vi "GetIQ_sglwfm.vi"(8 "error in (no error)":errorcluster, 11 "reference in":refnum<class "IQBurst_memo.lvclass">) -> (0 "error out":errorcluster, 2 "IQ":waveform(csg), 3 "reference out":refnum<class "IQBurst_memo.lvclass">)   [LabVIEW 2019, in "IQBurst_memo.lvclass"]
doc: "Return IQ data"
uses:
  IQBurst_memo.lvclass
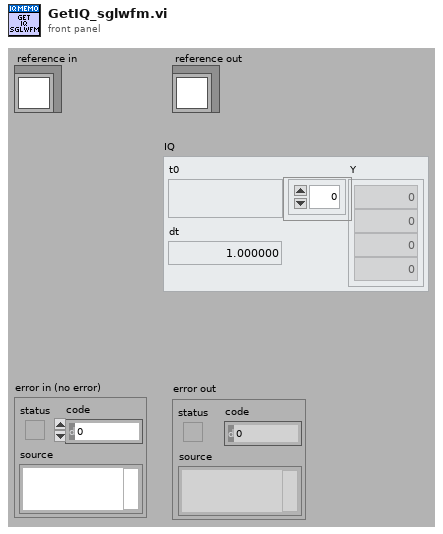
[diagram p1: front panel]
types:
  T1 = typedef "IQBurst_memo.lvclass/ObjectAttributes.ctl" = cluster{"IQ data":i16[], "dt":dbl}
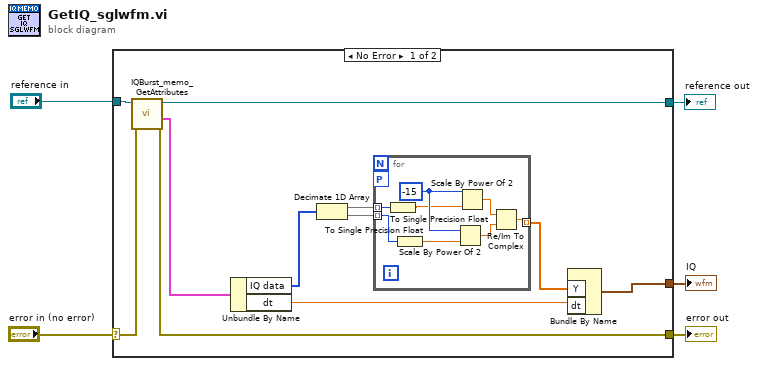
[diagram p0: block diagram]
diagram:
  n1 = case shown="No Error" "error in (no error)" {
    selector: "error in (no error)" -> [w16 w26]
    tunnel: [w15 w26] -> w4
    tunnel: [w14 w25] -> w2
    tunnel: "reference in" -> [w12 w25]
    tunnel: [w11 _] -> w1
    frame No Error {
      n2 = call "IQBurst_memo_GetAttributes.vi"("error in (no error)"=w16, "reference in"=w12) -> ("error out"=w15:errorcluster, "attributes"=w13:T1, "reference out"=w14:refnum<class "IQBurst_memo.lvclass">)  [unwired: 6 in, 1 out]
      n3 = Unbundle By Name(w13) -> ("IQ data"=w9:i16[], "dt"=w10:dbl)
      n4 = Decimate 1D Array(w9) -> (w8:i16[], w7:i16[])
      n5 = for {
        tunnel: w8 -> [w24] mode=indexing
        tunnel: w7 -> [w23] mode=indexing
        tunnel: [w17] -> w6 mode=indexing
        workers-P: _ -> [_]
        w22 = i16 -15 ("n")
        n6 = To Single Precision Float(number=w24) -> (single precision float=w21:sgl)
        n7 = To Single Precision Float(number=w23) -> (single precision float=w20:sgl)
        n8 = Scale By Power Of 2(n=w22, x=w20) -> (x*2^n=w18:sgl)
        n9 = Scale By Power Of 2(n=w22, x=w21) -> (x*2^n=w19:sgl)
        n10 = Re/Im To Complex(1:w18, 2:w19) -> (0:w17:csg)
      }
      n11 = Bundle By Name("Y"=w6, "dt"=w10) -> (w11:waveform(csg))  [unwired: 1 in]
    }
    frame Error {
    }
  }
  "error out" <- w4
  "reference out" <- w2
  "IQ" <- w1
